vi "backwards difference (i32).vi"(3 "Y":i32[](array[numeric])) -> (1 "Y(i)-Y(i-1)":i32[](array[numeric]))   [LabVIEW 2009, in "common.lvlib"]
uses:
  common.lvlib
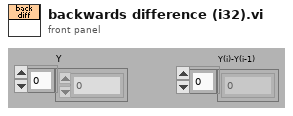
[diagram p1: front panel]
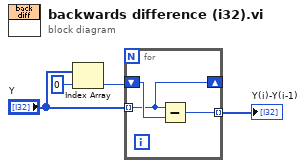
[diagram p0: block diagram]
diagram:
  n1 = Index Array(array="Y", index=0) -> (element=w2:i32)
  n2 = for {
    tunnel: "Y" -> [w6] mode=indexing
    shift-right: [w6] -> _
    shift-left: w2 -> [w7]
    tunnel: [w5] -> w1 mode=indexing
    n3 = Subtract(x=w6, y=w7) -> (x-y=w5:i32)
  }
  "Y(i)-Y(i-1)" <- w1
